vi "주차 알고리즘.vi"() -> ()   [LabVIEW 2016]
uses:
  <vilib>/imath/engines/lvmath2/RunTimeEngine/Managers/WorkSpace/UID Generator.vi
  <vilib>/imath/engines/lvmath2/RunTimeEngine/BuiltInFunctions/size/NIMS_I32Row=size(GM).vi
  <instcachedir>/0/NIMS_I32Row=size(GM)_10ACDCB9F1F84A7E9F42C91D87611FB5.lvgen/NIMS_I32Row=size(GM)_10ACDCB9F1F84A7E9F42C91D87611FB5_001.vi
  <vilib>/imath/engines/lvmath2/RunTimeEngine/RunTimeType/NIMS_RunTimeType_From StrictType (excl LVString).vi
  <instcachedir>/0/NIMS_RunTimeType_From StrictType (excl LVString)_BBF44FB49F834B71AF7A14CCEDF8BECD.lvgen/NIMS_RunTimeType_From StrictType (excl LVString)_BBF44FB49F834B71AF7A14CCEDF8BECD_000.vi
  <vilib>/imath/engines/lvmath2/RunTimeEngine/LocalVariableDefStatement/MC_LocalVariableDefStatement_Display.vi
  <vilib>/imath/engines/lvmath2/RunTimeEngine/IndexRead/NIMS V(S).vi
  <instcachedir>/0/NIMS V(S)_0488751826AF41519A22953C041130DC.lvgen/NIMS V(S)_0488751826AF41519A22953C041130DC_002.vi
  <vilib>/imathl/engines/lvmath/Functions/Error Handling/Create Error.vi
  <vilib>/imath/engines/lvmath2/RunTimeEngine/Managers/SymbolTable/Clear UID.vi
  <vilib>/imath/engines/lvmath2/RunTimeEngine/NodeEndStatement/NIMS_NodeEndStatement_Output.vi
  <instcachedir>/0/NIMS_NodeEndStatement_Output_53EC0D466D134D7ABD903AC30B43404B.lvgen/NIMS_NodeEndStatement_Output_53EC0D466D134D7ABD903AC30B43404B_011.vi
  <vilib>/imath/engines/lvmath2/RunTimeEngine/ErrorHandling/NIMS_Finalize Error.vi
  <vilib>/imath/engines/lvmath2/RunTimeEngine/Managers/SymbolTable/NIMS_WorkSpace.lvlib
panel:
  out "p5":dbl
  out "p4":dbl
  out "p3":dbl
  out "p2":dbl
  out "시작포인트 2":dbl
  out "Brake":i16
  out "Platform Speed":i16
  out "시작포인트":dbl
  in  "encoder":dbl
  out "에러 출력":errorcluster
  in  "filter angle(end)":dbl
  in  "filter angle(start)":dbl
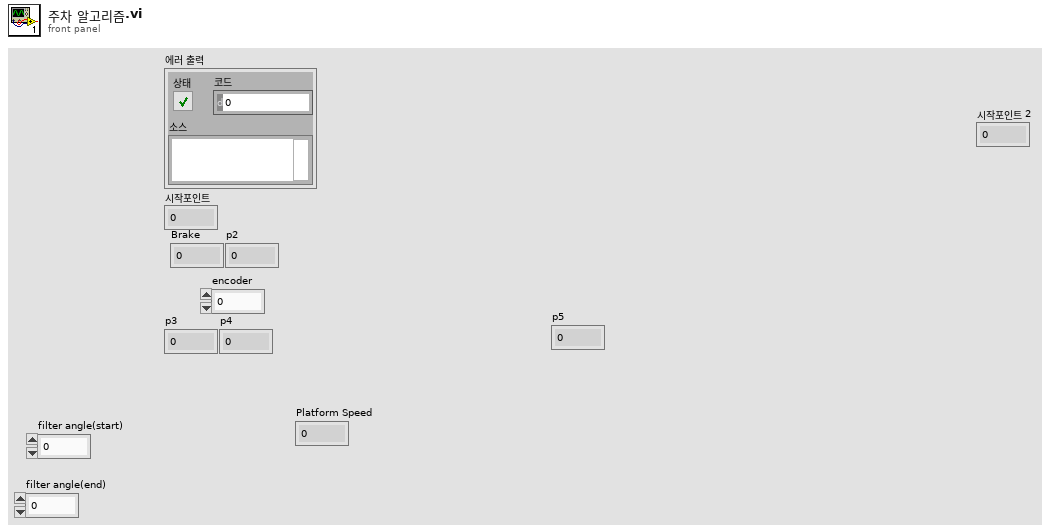
[diagram p1: front panel]
types:
  T1 = typedef "2차원배열 공유변수.ctl" = dbl[][]
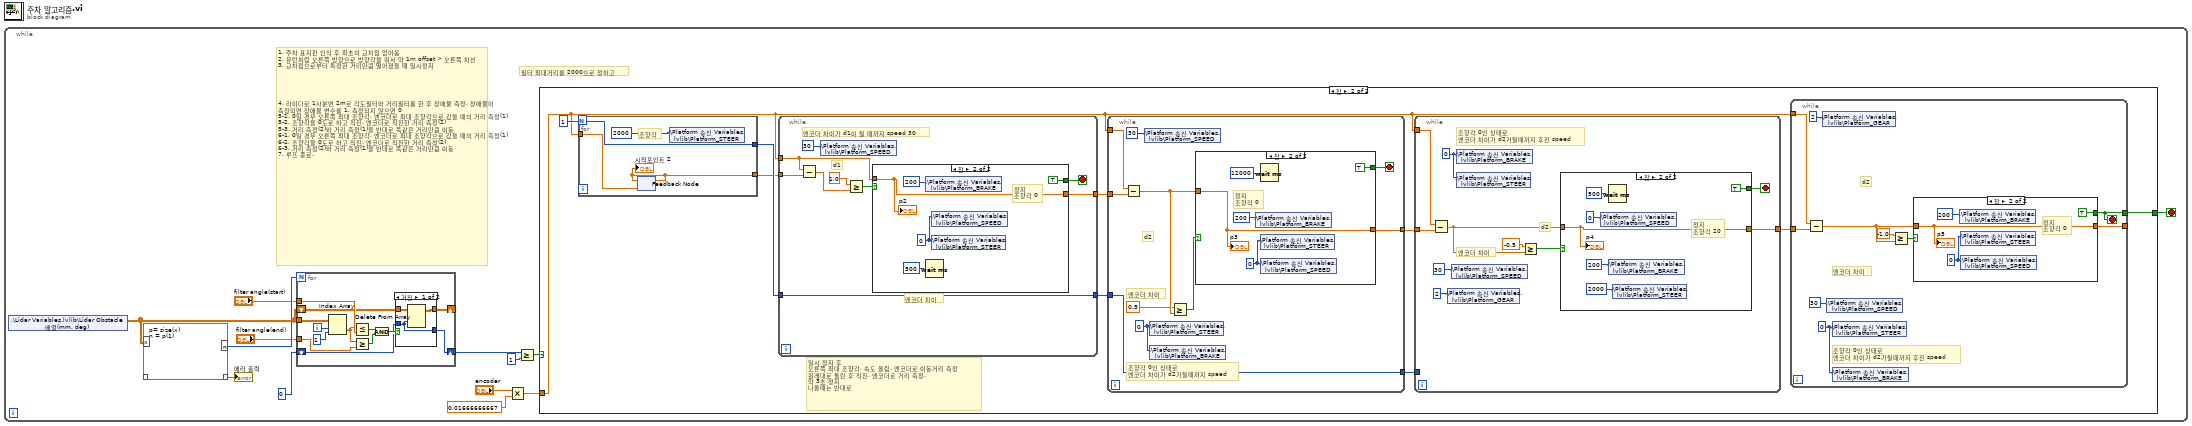
[diagram p0: block diagram]
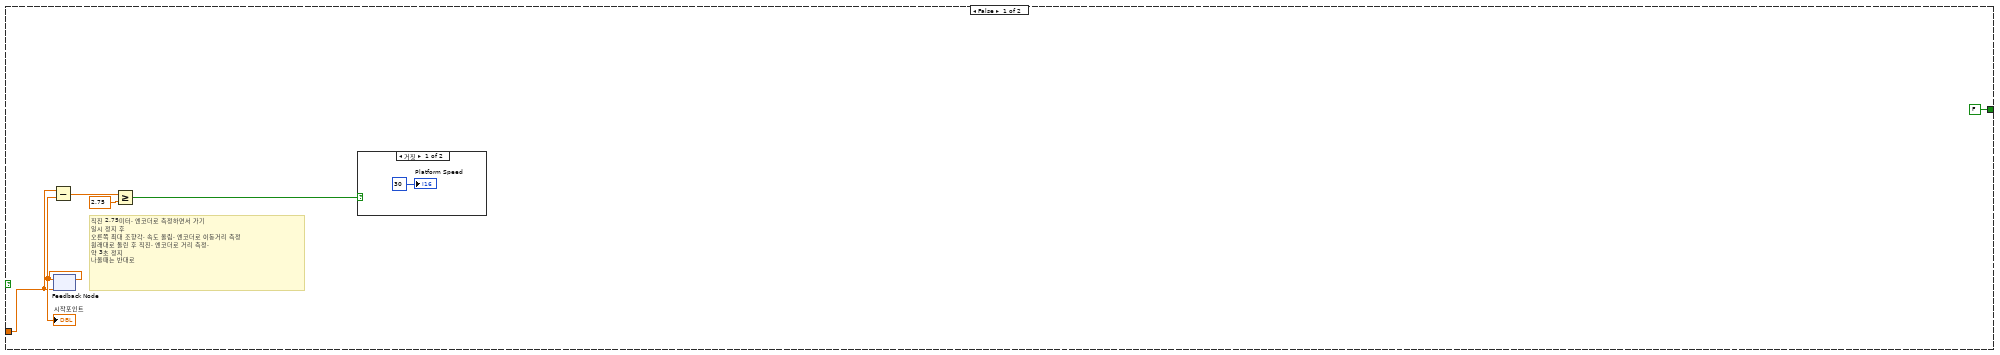
[diagram p2: hidden frame]
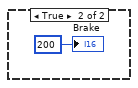
[diagram p3: hidden frame]
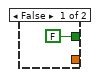
[diagram p4: hidden frame]
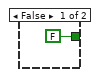
[diagram p5: hidden frame]
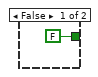
[diagram p6: hidden frame]
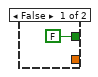
[diagram p7: hidden frame]
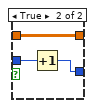
[diagram p8: hidden frame]
diagram:
  n1 = while {
    stop <- w2 stop-if-true
    # "필터 최대거리를 2000으로 정하고"
    # "1. 주차 표지판 인식 후 최초의 교차점 얻어옴\n2. 유턴처럼 오른쪽 방향으로 방향각을 줘서 약 1m offset > 오른쪽 차선\n3. 교차점으로부터 특정한 거리만큼 떨어졌을 때 일시정지\n\n\n\n\n\n4. 라이다로 1사분면 2m로 각도필터와 거리필터를 한 후 장애물 측정. 장애물이 측정되면 장애물 변수를 1, 측정되지 않으면 0\n5-1. 0일 경우 오른쪽 최대 조향각. 엔코더로 최대 조향각으로 갔을 때의 거리 측정(1)\n5-2. 조향각을 0도로 하고 직진. 엔코더로 직진한 거리 측정(2)\n5-3. 거리 측정(2)와 거리 측정(1)을 반대로 똑같은 거리만큼 이동\n6-1. 0일 경우 오른쪽 최대 조향각. 엔코더로 최대 조향각으로 갔을 때의 거리 측정(1)\n6-2. 조향각을 0도로 하고 직진. 엔코더로 직진한 거리 측정(2)\n6-3. 거리 측정(2)와 거리 측정(1)을 반대로 똑같은 거리만큼 이동\n7. 루프 종료."
    n2 = shared-variable ".\\Lidar Variables.lvlib\\Lidar Obstacle 배열(mm, deg)"() -> (w1:T1)  [unwired: 1 in, 1 out]
    n3 = mathscript code="p= size(x)\nn = p(1)"("x"=w1) -> ("??"=→"에러 출력":errorcluster, "n"=w13:i32)  [unwired: 1 in]
    n4 = for {
      N: w13 -> [_]
      tunnel: "filter angle(start)" -> [w172]
      tunnel: "filter angle(end)" -> [w170]
      shift-right: [w163] -> w8
      shift-left: 0 ("비활성화된 인덱스 (행)") -> [w165]
      shift-right: [w164] -> _
      shift-left: w1 -> [w166]
      tunnel: w1 -> [w162]
      i -> [w161]
      n5 = Index Array(array=w162, index (row)=w161, index (col)=1 ("비활성화된 인덱스 (열)")) -> (element=w171:dbl)
      n6 = Less Or Equal?(x=w171, y=w172) -> (x <= y?=w169:bool)
      n7 = Greater Or Equal?(x=w171, y=w170) -> (x >= y?=w168:bool)
      n8 = And(x=w169, y=w168) -> (x .and. y?=w167:bool)
      n9 = case shown="거짓" w167 {
        tunnel: w166 -> [w176 w177]
        tunnel: w165 -> [w174 w179]
        tunnel: [w175 w177] -> w164
        tunnel: [w174 w178] -> w163
        frame False {
          n10 = Delete From Array(array=w176, index (row)=w174) -> (array with subset deleted=w175:T1)  [unwired: 2 in, 1 out]
        }
        frame True {
          n11 = Increment(x=w179) -> (x+1=w178:i32)
        }
      }
    }
    n12 = Multiply(x="encoder", y=0.01666666667) -> (x*y=w3:dbl)
    n13 = Greater Or Equal?(x=w8, y=1) -> (x >= y?=w6:bool)
    n14 = case shown="참" w6 {
      tunnel: w3 -> [w15 w23]
      tunnel: [FALSE w22] -> w2
      frame False {
        # "직진 2.75미터. 엔코더로 측정하면서 가기\n일시 정지 후 \n오른쪽 최대 조향각, 속도 올림. 엔코더로 이동거리 측정\n원래대로 돌린 후 직진. 엔코더로 거리 측정.\n약 3초 정지\n나올때는 반대로"
        n15 = feedback #1(w15) -> (w19:dbl)
        "시작포인트" <- w19
        n16 = Subtract(x=w15, y=w19) -> (x-y=w18:dbl)
        n17 = feedback-in #1(w19) -> ()
        n18 = Greater Or Equal?(x=w18, y=2.75) -> (x >= y?=w16:bool)
        n19 = case shown="거짓" w16 {
          frame False {
            "Platform Speed" <- i16 30 ("Platform Speed")
          }
          frame True {
            "Brake" <- i16 200 ("Brake")
          }
        }
      }
      frame True {
        # "일시 정지 후 \n오른쪽 최대 조향각, 속도 올림. 엔코더로 이동거리 측정\n원래대로 돌린 후 직진. 엔코더로 거리 측정.\n약 3초 정지\n나올때는 반대로"
        n20 = for {
          N: 1 -> [w97]
          tunnel: w23 -> [w98]
          tunnel: [w97] -> w30
          tunnel: [w96] -> w27
          # "조향각"
          n21 = feedback #2(w98) -> (w96:dbl)
          "시작포인트 2" <- w96
          n22 = feedback-in #2(w96) -> ()
          n23 = shared-variable ".\\Platform 송신 Variables.lvlib\\Platform_STEER"(i16 2000) -> ()  [unwired: 1 in, 1 out]
        }
        n24 = while {
          tunnel: [w87] -> w29
          tunnel: w30 -> [w87]
          tunnel: w23 -> [w82]
          tunnel: w27 -> [w85]
          tunnel: [w81] -> w26
          stop <- w86 stop-if-true
          # "d1"
          # "엔코더 차이"
          # "엔코더 차이가 d1이 될 때까지 speed 30"
          n25 = Subtract(x=w82, y=w85) -> (x-y=w84:dbl)
          n26 = shared-variable ".\\Platform 송신 Variables.lvlib\\Platform_SPEED"(i16 30) -> ()  [unwired: 1 in, 1 out]
          n27 = Greater Or Equal?(x=1.0, y=w84) -> (x >= y?=w88:bool)
          n28 = case shown="참" w88 {
            tunnel: [FALSE TRUE] -> w86
            tunnel: w82 -> [_ w92]
            tunnel: [_ w92] -> w81
            frame False {
            }
            frame True {
              w91 = i16 0
              # "정지\n조향각 0"
              n29 = shared-variable ".\\Platform 송신 Variables.lvlib\\Platform_BRAKE"(i16 200) -> ()  [unwired: 1 in, 1 out]
              n30 = Wait (ms)(milliseconds to wait=u32 500 ("대기 시간 (ms)")) -> ()  [unwired: 1 out]
              n31 = shared-variable ".\\Platform 송신 Variables.lvlib\\Platform_SPEED"(w91) -> ()  [unwired: 1 in, 1 out]
              n32 = shared-variable ".\\Platform 송신 Variables.lvlib\\Platform_STEER"(w91) -> ()  [unwired: 1 in, 1 out]
              "p2" <- w92
            }
          }
        }
        n33 = while {
          tunnel: w29 -> [w71]
          tunnel: [w71] -> w28
          tunnel: w26 -> [w70]
          tunnel: w23 -> [w69]
          tunnel: [w67] -> w25
          stop <- w72 stop-if-true
          w65 = i16 0
          # "d2"
          # "엔코더 차이"
          # "조향각 0인 상태로\n엔코더 차이가 d2가될때까지 speed"
          n34 = Subtract(x=w69, y=w70) -> (x-y=w68:dbl)
          n35 = shared-variable ".\\Platform 송신 Variables.lvlib\\Platform_SPEED"(i16 30) -> ()  [unwired: 1 in, 1 out]
          n36 = shared-variable ".\\Platform 송신 Variables.lvlib\\Platform_STEER"(w65) -> ()  [unwired: 1 in, 1 out]
          n37 = shared-variable ".\\Platform 송신 Variables.lvlib\\Platform_BRAKE"(w65) -> ()  [unwired: 1 in, 1 out]
          n38 = Greater Or Equal?(x=0.5, y=w68) -> (x >= y?=w73:bool)
          n39 = case shown="참" w73 {
            tunnel: [FALSE TRUE] -> w72
            tunnel: w68 -> [_ w77]
            tunnel: [_ w77] -> w67
            frame False {
            }
            frame True {
              w75 = i16 0
              # "정지\n조향각 0"
              n40 = shared-variable ".\\Platform 송신 Variables.lvlib\\Platform_BRAKE"(i16 200) -> ()  [unwired: 1 in, 1 out]
              n41 = Wait (ms)(milliseconds to wait=u32 12000 ("대기 시간 (ms)")) -> ()  [unwired: 1 out]
              n42 = shared-variable ".\\Platform 송신 Variables.lvlib\\Platform_STEER"(w75) -> ()  [unwired: 1 in, 1 out]
              n43 = shared-variable ".\\Platform 송신 Variables.lvlib\\Platform_SPEED"(w75) -> ()  [unwired: 1 in, 1 out]
              "p3" <- w77
            }
          }
        }
        n44 = while {
          tunnel: w28 -> [_]
          tunnel: w23 -> [w54]
          tunnel: w25 -> [w53]
          tunnel: [w50] -> w24
          stop <- w55 stop-if-true
          w49 = i16 0
          # "d2"
          # "엔코더 차이"
          # "조향각 0인 상태로\n엔코더 차이가 d2가될때까지 후진 speed"
          n45 = Subtract(x=w54, y=w53) -> (x-y=w51:dbl)
          n46 = shared-variable ".\\Platform 송신 Variables.lvlib\\Platform_GEAR"(i16 2 ("Gear")) -> ()  [unwired: 1 in, 1 out]
          n47 = shared-variable ".\\Platform 송신 Variables.lvlib\\Platform_SPEED"(i16 30) -> ()  [unwired: 1 in, 1 out]
          n48 = shared-variable ".\\Platform 송신 Variables.lvlib\\Platform_BRAKE"(w49) -> ()  [unwired: 1 in, 1 out]
          n49 = shared-variable ".\\Platform 송신 Variables.lvlib\\Platform_STEER"(w49) -> ()  [unwired: 1 in, 1 out]
          n50 = Greater Or Equal?(x=-0.5, y=w51) -> (x >= y?=w56:bool)
          n51 = case shown="참" w56 {
            tunnel: [FALSE TRUE] -> w55
            tunnel: w51 -> [_ w62]
            tunnel: [_ w62] -> w50
            frame False {
            }
            frame True {
              # "정지\n조향각 20"
              n52 = shared-variable ".\\Platform 송신 Variables.lvlib\\Platform_SPEED"(i16 0) -> ()  [unwired: 1 in, 1 out]
              n53 = Wait (ms)(milliseconds to wait=u32 500 ("대기 시간 (ms)")) -> ()  [unwired: 1 out]
              n54 = shared-variable ".\\Platform 송신 Variables.lvlib\\Platform_BRAKE"(i16 200) -> ()  [unwired: 1 in, 1 out]
              n55 = shared-variable ".\\Platform 송신 Variables.lvlib\\Platform_STEER"(i16 2000 ("Platform_STEER")) -> ()  [unwired: 1 in, 1 out]
              "p4" <- w62
            }
          }
        }
        n56 = while {
          tunnel: w23 -> [w40]
          tunnel: w24 -> [w39]
          tunnel: [w36] -> _
          tunnel: [w35] -> w22
          stop <- w35 stop-if-true
          w33 = i16 0
          # "d2"
          # "엔코더 차이"
          # "조향각 0인 상태로\n엔코더 차이가 d2가될때까지 후진 speed"
          n57 = Subtract(x=w40, y=w39) -> (x-y=w37:dbl)
          n58 = shared-variable ".\\Platform 송신 Variables.lvlib\\Platform_GEAR"(i16 2 ("Gear")) -> ()  [unwired: 1 in, 1 out]
          n59 = shared-variable ".\\Platform 송신 Variables.lvlib\\Platform_SPEED"(i16 30) -> ()  [unwired: 1 in, 1 out]
          n60 = shared-variable ".\\Platform 송신 Variables.lvlib\\Platform_STEER"(w33) -> ()  [unwired: 1 in, 1 out]
          n61 = shared-variable ".\\Platform 송신 Variables.lvlib\\Platform_BRAKE"(w33) -> ()  [unwired: 1 in, 1 out]
          n62 = Greater Or Equal?(x=-1.0, y=w37) -> (x >= y?=w41:bool)
          n63 = case shown="참" w41 {
            tunnel: [FALSE TRUE] -> w35
            tunnel: w37 -> [_ w45]
            tunnel: [_ w45] -> w36
            frame False {
            }
            frame True {
              w44 = i16 0
              # "정지\n조향각 0"
              n64 = shared-variable ".\\Platform 송신 Variables.lvlib\\Platform_BRAKE"(i16 200) -> ()  [unwired: 1 in, 1 out]
              n65 = shared-variable ".\\Platform 송신 Variables.lvlib\\Platform_STEER"(w44) -> ()  [unwired: 1 in, 1 out]
              n66 = shared-variable ".\\Platform 송신 Variables.lvlib\\Platform_SPEED"(w44) -> ()  [unwired: 1 in, 1 out]
              "p5" <- w45
            }
          }
        }
      }
    }
  }
